vi "DSF.Engine.Memory.Cache.Transfer.Get Largest Count.All Types.vi"(8 "error in (no error)":errorcluster, 10 "Data Type Counts in":T1 {"U64" format="%d elements"; "U32" format="%d elements"; "U16" format="%d elements"; "U8" format="%d elements"; "I64" format="%d elements"; "I32" format="%d elements"; "I16" format="%d elements"; "I8" format="%d elements"; "DBL" format="%d elements"; "SGL" format="%d elements"; "Bool" format="%d elements"}, 11 "Transfer Cache in":refnum<class "DSF.Engine.Memory.Cache.Transfer.lvclass">) -> (0 "error out":errorcluster, 2 "Data Type Counts out":T1 {"U64" format="%d elements"; "U32" format="%d elements"; "U16" format="%d elements"; "U8" format="%d elements"; "I64" format="%d elements"; "I32" format="%d elements"; "I16" format="%d elements"; "I8" format="%d elements"; "DBL" format="%d elements"; "SGL" format="%d elements"; "Bool" format="%d elements"}, 3 "Transfer Cache out":refnum<class "DSF.Engine.Memory.Cache.Transfer.lvclass">)   [LabVIEW 2017, in "DSF.Engine.lvlib" / "DSF.Engine.Memory.Cache.Transfer.lvclass"]
uses:
  DSF.Engine.Memory.Cache.Transfer.lvclass
  Shared/Classes/Transfer/DSF.Shared.Configuration.Transfer.lvclass
  Shared/Typedefs/DSF.Shared.Typedefs.Data Type Counts.ctl
  DSF.Shared.lvlib
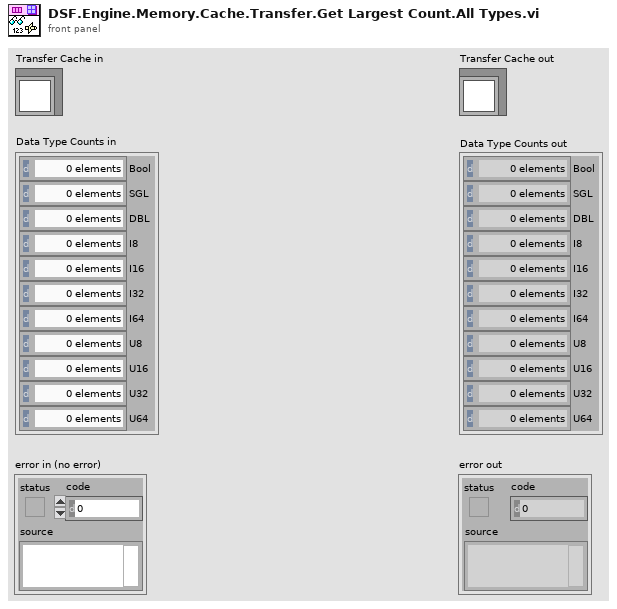
[diagram p1: front panel]
types:
  T1 = typedef "DSF.Shared.lvlib/DSF.Shared.Typedefs.Data Type Counts.ctl" = cluster{"Bool":u64, "SGL":u64, "DBL":u64, "I8":u64, "I16":u64, "I32":u64, "I64":u64, "U8":u64, "U16":u64, "U32":u64, "U64":u64}
  T2 = typedef "DSF.Shared.lvlib/DSF.Shared.Typedefs.Configuration.Transfer.Channel Block Descriptor.ctl" = cluster{"First Channel Descriptor":T3, "count":u64, "vs channel index":u64}
  T3 = typedef "DSF.Shared.lvlib/DSF.Shared.Typedefs.Configuration.Transfer.Channel Descriptor.ctl" = cluster{"Channel Parameters":T4, "VS Channel Ref":T6}
  T4 = typedef "DSF.Shared.lvlib/DSF.Shared.Typedefs.Configuration.Transfer.Channel Parameters.ctl" = cluster{"offset":u64, "data type":T5}
  T5 = typedef "DSF.Shared.lvlib/DSF.Shared.Typedefs.Data Type.ctl" = enum8{"Bool", "SGL", "DBL", "I8", "I16", "I32", "I64", "U8", "U16", "U32", "U64"}
  T6 = typedef "Custom Device API.lvlib/Custom Device Item Ref.ctl" = u64
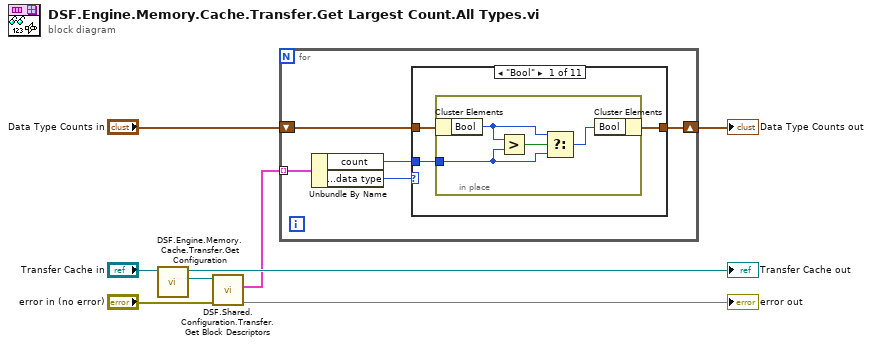
[diagram p0: block diagram]
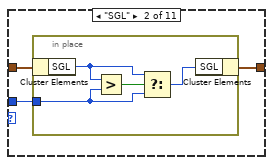
[diagram p2: hidden frame]
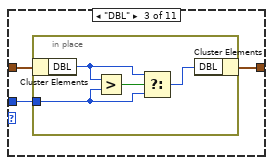
[diagram p3: hidden frame]
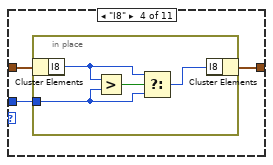
[diagram p4: hidden frame]
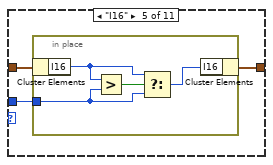
[diagram p5: hidden frame]
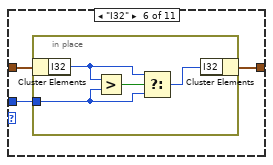
[diagram p6: hidden frame]
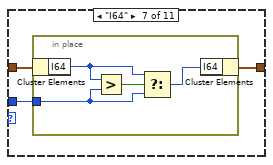
[diagram p7: hidden frame]
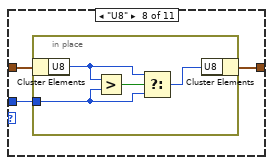
[diagram p8: hidden frame]
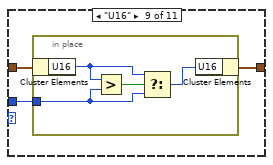
[diagram p9: hidden frame]
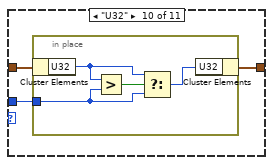
[diagram p10: hidden frame]
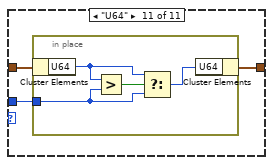
[diagram p11: hidden frame]
diagram:
  n1 = call "DSF.Engine.Memory.Cache.Transfer.Get Configuration.vi"("Transfer Cache in"="Transfer Cache in") -> ("Transfer Configuration"=w4:refnum<class "DSF.Shared.Configuration.Transfer.lvclass">, "Transfer Cache out"=→"Transfer Cache out":refnum<class "DSF.Engine.Memory.Cache.Transfer.lvclass">)  [unwired: 9 in]
  n2 = call "DSF.Shared.Configuration.Transfer.Get Block Descriptors.vi"(8:"error in (no error)", "Transfer Configuration in"=w4) -> (0:→"error out", "Channel Blocks"=w2:T2[])  [unwired: 7 in, 1 out]
  n3 = for {
    tunnel: w2 -> [w13] mode=indexing
    shift-right: [w9] -> w7
    shift-left: "Data Type Counts in" -> [w11]
    n4 = Unbundle By Name(w13) -> ("count"=w10:u64, "First Channel Descriptor.Channel Parameters.data type"=w12:T5)
    n5 = case shown="\"Bool\"" w12 {
      tunnel: w11 -> [w16 w23 w30 w37 w44 w51 w58 w65 w72 w79 w86]
      tunnel: w10 -> [w15 w22 w29 w36 w43 w50 w57 w64 w71 w78 w85]
      tunnel: [w14 w21 w28 w35 w42 w49 w56 w63 w70 w77 w84] -> w9
      frame "Bool" {
        n6 = in-place {
          in-place-border: w15 -> [w18]
          n7 = in-place-cluster #1(w16) -> ("Bool"=w19:u64)
          n8 = Greater?(x=w19, y=w18) -> (0:w20:bool)
          n9 = Select(t=w19, s=w20, f=w18) -> (s? t:f=w17:u64)
          n10 = in-place-cluster #1("Bool"=w17) -> (w14:T1)
        }
      }
      frame "SGL" {
        n11 = in-place {
          in-place-border: w22 -> [w25]
          n12 = in-place-cluster #2(w23) -> ("SGL"=w26:u64)
          n13 = Greater?(x=w26, y=w25) -> (0:w27:bool)
          n14 = Select(t=w26, s=w27, f=w25) -> (s? t:f=w24:u64)
          n15 = in-place-cluster #2("SGL"=w24) -> (w21:T1)
        }
      }
      frame "DBL" {
        n16 = in-place {
          in-place-border: w29 -> [w32]
          n17 = in-place-cluster #3(w30) -> ("DBL"=w33:u64)
          n18 = Greater?(x=w33, y=w32) -> (0:w34:bool)
          n19 = Select(t=w33, s=w34, f=w32) -> (s? t:f=w31:u64)
          n20 = in-place-cluster #3("DBL"=w31) -> (w28:T1)
        }
      }
      frame "I8" {
        n21 = in-place {
          in-place-border: w36 -> [w39]
          n22 = in-place-cluster #4(w37) -> ("I8"=w40:u64)
          n23 = Greater?(x=w40, y=w39) -> (0:w41:bool)
          n24 = Select(t=w40, s=w41, f=w39) -> (s? t:f=w38:u64)
          n25 = in-place-cluster #4("I8"=w38) -> (w35:T1)
        }
      }
      frame "I16" {
        n26 = in-place {
          in-place-border: w43 -> [w46]
          n27 = in-place-cluster #5(w44) -> ("I16"=w47:u64)
          n28 = Greater?(x=w47, y=w46) -> (0:w48:bool)
          n29 = Select(t=w47, s=w48, f=w46) -> (s? t:f=w45:u64)
          n30 = in-place-cluster #5("I16"=w45) -> (w42:T1)
        }
      }
      frame "I32" {
        n31 = in-place {
          in-place-border: w50 -> [w53]
          n32 = in-place-cluster #6(w51) -> ("I32"=w54:u64)
          n33 = Greater?(x=w54, y=w53) -> (0:w55:bool)
          n34 = Select(t=w54, s=w55, f=w53) -> (s? t:f=w52:u64)
          n35 = in-place-cluster #6("I32"=w52) -> (w49:T1)
        }
      }
      frame "I64" {
        n36 = in-place {
          in-place-border: w57 -> [w60]
          n37 = in-place-cluster #7(w58) -> ("I64"=w61:u64)
          n38 = Greater?(x=w61, y=w60) -> (0:w62:bool)
          n39 = Select(t=w61, s=w62, f=w60) -> (s? t:f=w59:u64)
          n40 = in-place-cluster #7("I64"=w59) -> (w56:T1)
        }
      }
      frame "U8" {
        n41 = in-place {
          in-place-border: w64 -> [w67]
          n42 = in-place-cluster #8(w65) -> ("U8"=w68:u64)
          n43 = Greater?(x=w68, y=w67) -> (0:w69:bool)
          n44 = Select(t=w68, s=w69, f=w67) -> (s? t:f=w66:u64)
          n45 = in-place-cluster #8("U8"=w66) -> (w63:T1)
        }
      }
      frame "U16" {
        n46 = in-place {
          in-place-border: w71 -> [w74]
          n47 = in-place-cluster #9(w72) -> ("U16"=w75:u64)
          n48 = Greater?(x=w75, y=w74) -> (0:w76:bool)
          n49 = Select(t=w75, s=w76, f=w74) -> (s? t:f=w73:u64)
          n50 = in-place-cluster #9("U16"=w73) -> (w70:T1)
        }
      }
      frame "U32" {
        n51 = in-place {
          in-place-border: w78 -> [w81]
          n52 = in-place-cluster #10(w79) -> ("U32"=w82:u64)
          n53 = Greater?(x=w82, y=w81) -> (0:w83:bool)
          n54 = Select(t=w82, s=w83, f=w81) -> (s? t:f=w80:u64)
          n55 = in-place-cluster #10("U32"=w80) -> (w77:T1)
        }
      }
      frame "U64" {
        n56 = in-place {
          in-place-border: w85 -> [w88]
          n57 = in-place-cluster #11(w86) -> ("U64"=w89:u64)
          n58 = Greater?(x=w89, y=w88) -> (0:w90:bool)
          n59 = Select(t=w89, s=w90, f=w88) -> (s? t:f=w87:u64)
          n60 = in-place-cluster #11("U64"=w87) -> (w84:T1)
        }
      }
    }
  }
  "Data Type Counts out" <- w7
